vi "Write Controller Enqueuer.vi"(10 "Actor Framework:Message Enqueuer":refnum<class "Message Enqueuer.lvclass">, 11 "User Interface in":refnum<class "User Interface.lvclass">) -> (3 "User Interface out":refnum<class "User Interface.lvclass">)   [LabVIEW 2016, in "_User Interface.lvlib" / "User Interface.lvclass"]
uses:
  User Interface.lvclass
  <vilib>/ActorFramework/Message Enqueuer/Message Enqueuer.lvclass
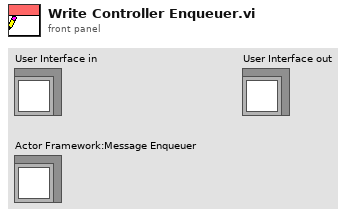
[diagram p1: front panel]
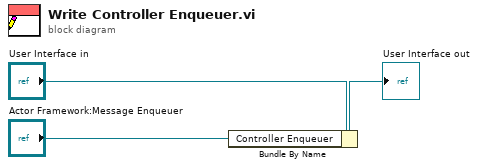
[diagram p0: block diagram]
diagram:
  n1 = Bundle By Name(cluster="User Interface in", "Controller Enqueuer"="Actor Framework:Message Enqueuer") -> (→"User Interface out":refnum<class "User Interface.lvclass">)
